vi "LabVIEW own project.vi"() -> ()   [LabVIEW 2025]
uses:
  <vilib>/measure/NI_MABase.lvlib
panel:
  in  "Boolean":bool
  in  "amplitude 3":dbl=1.0 format="%0.2p"
  in  "frequency 3":dbl=10.0 format="%0.2p"
  in  "amplitude 2":dbl=1.0 format="%0.2p"
  in  "frequency 2":dbl=10.0 format="%0.2p"
  out "Waveform Chart":waveform(dbl)(graph)
  in  "amplitude":dbl=1.0 format="%0.2p"
  in  "frequency":dbl=10.0 format="%0.2p"
  in  "stop":bool
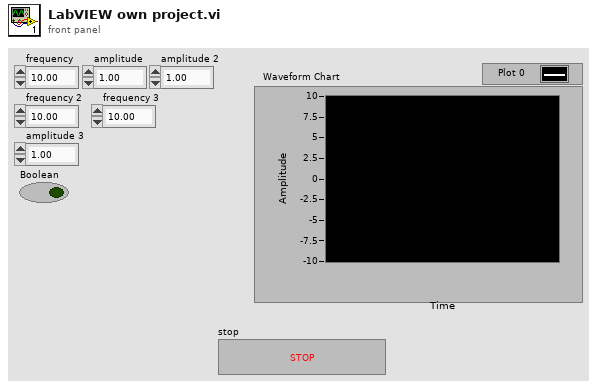
[diagram p1: front panel]
types:
  T1 = enum16{"Sine Wave", "Triangle Wave", "Square Wave", "Sawtooth Wave"}
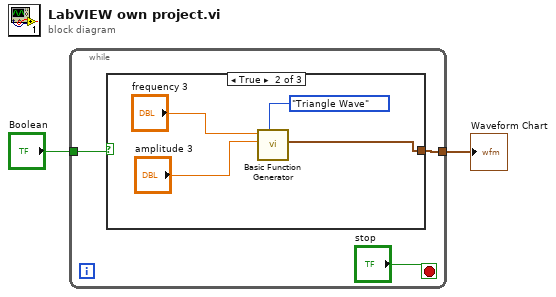
[diagram p0: block diagram]
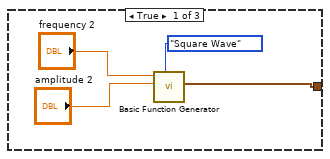
[diagram p2: hidden frame]
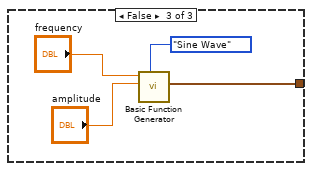
[diagram p3: hidden frame]
diagram:
  n1 = while {
    tunnel: [w4] -> w2
    tunnel: "Boolean" -> [w3]
    stop <- "stop" stop-if-true
    n2 = case shown="\"Triangle\"" w3 {
      tunnel: [w7 w11 w15] -> w4
      frame True {
        n3 = call <vilib>:"Basic Function Generator.vi"("signal type"=T1."Square Wave", "amplitude"="amplitude 2", "frequency"="frequency 2") -> ("signal out"=w7:waveform(dbl))  [unwired: 6 in, 2 out]
      }
      frame True {
        n4 = call <vilib>:"Basic Function Generator.vi"("signal type"=T1."Triangle Wave", "amplitude"="amplitude 3", "frequency"="frequency 3") -> ("signal out"=w11:waveform(dbl))  [unwired: 6 in, 2 out]
      }
      frame False {
        n5 = call <vilib>:"Basic Function Generator.vi"("signal type"=T1."Sine Wave", "amplitude"="amplitude", "frequency"="frequency") -> ("signal out"=w15:waveform(dbl))  [unwired: 6 in, 2 out]
      }
    }
  }
  "Waveform Chart" <- w2
